vi "HEWH_Ritter_GasMeter.vi"(8 "error in":errorcluster, 11 "Message Queues out":T1) -> (0 "error out":errorcluster)   [LabVIEW 2023]
uses:
  Tenney/support/Message Queue/All Message Queues.ctl
  Tenney/support/Message Queue/Message Cluster.ctl
  Drivers/Ritter Gas Meter/Type Definitions/Ritter Data.ctl
  FVIR and LDO/support/Message Queue/Enqueue Message (Single).vi
  FVIR and LDO/support/Message Queue/Message Queue.lvlib
  Tenney/support/Message Queue/Tenney Message Queue.lvlib
panel:
  out "Loop Count":i32
  in  "Debug":bool
  out "Debug":string[](array[string])
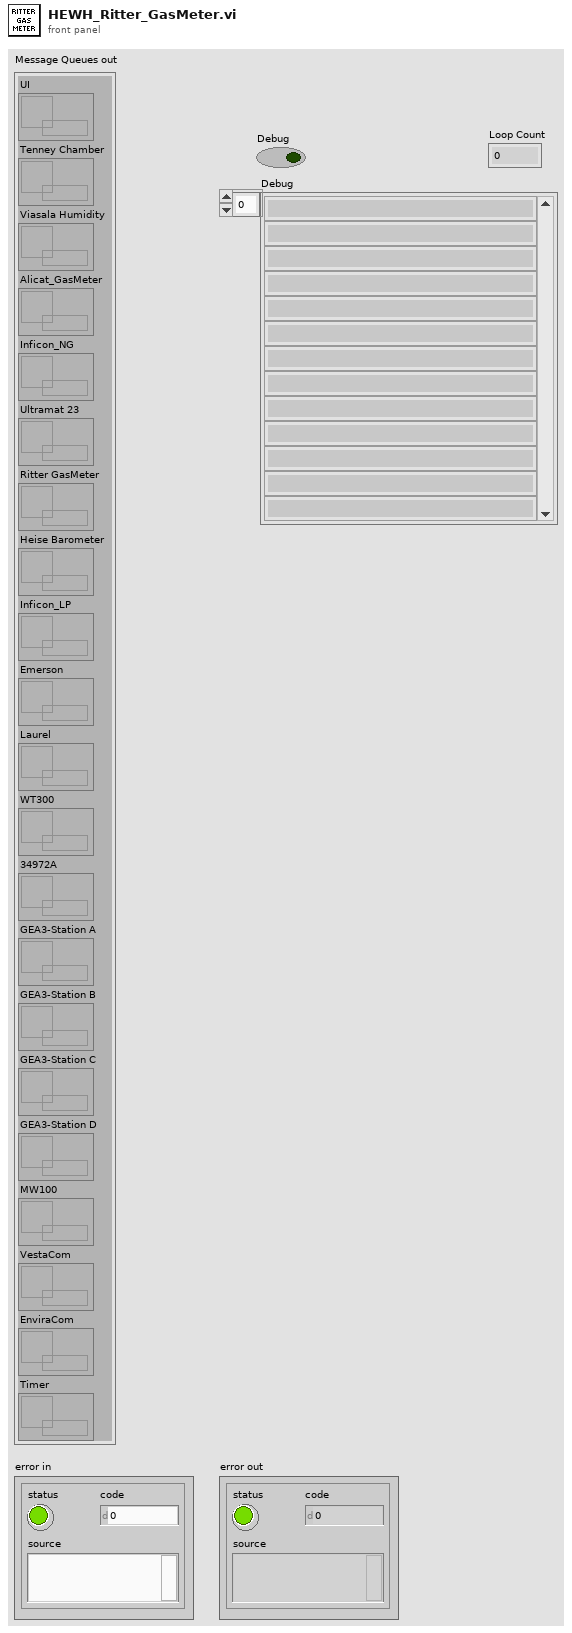
[diagram p1: front panel]
types:
  T1 = typedef "Tenney Message Queue.lvlib/All Message Queues.ctl" = cluster{"UI":refnum<queue>, "Tenney Chamber":refnum<queue>, "Viasala Humidity":refnum<queue>, "Alicat_GasMeter":refnum<queue>, "Inficon_NG":refnum<queue>, "Ultramat 23":refnum<queue>, "Ritter GasMeter":refnum<queue>, "Heise Barometer":refnum<queue>, "Inficon_LP":refnum<queue>, "Emerson":refnum<queue>, "Laurel":refnum<queue>, "WT300":refnum<queue>, "34972A":refnum<queue>, "GEA3-Station A":refnum<queue>, "GEA3-Station B":refnum<queue>, "GEA3-Station C":refnum<queue>, "GEA3-Station D":refnum<queue>, "MW100":refnum<queue>, "VestaCom":refnum<queue>, "EnviraCom":refnum<queue>, "Timer":refnum<queue>}
  T2 = typedef "Ritter Data.ctl" = cluster{"Gas Flow Rate (L/hr)-Uncorrected":dbl, "Totalized Flow (L)--Uncorrected":dbl, "Gas Flow Rate (cuft/hr)-Uncorrected":dbl, "Totalized Flow (cuft)-Uncorrected":dbl, "Gas Temperature (F)":dbl, "Gas Pressure (in WC)":dbl, "Heise Barometric Pressure (inHG)":dbl, "STP Correction Factor":dbl, "Temp Correction Factor":dbl, "Pressure Correction Factor":dbl, "Water Vapor Pressure":dbl, "Gas Flow Rate (cuft/hr)-Corrected":dbl, "Totalized Flow (cuft)-Corrected":dbl, "Gas BTU":dbl, "Gas BTU/hr":dbl}
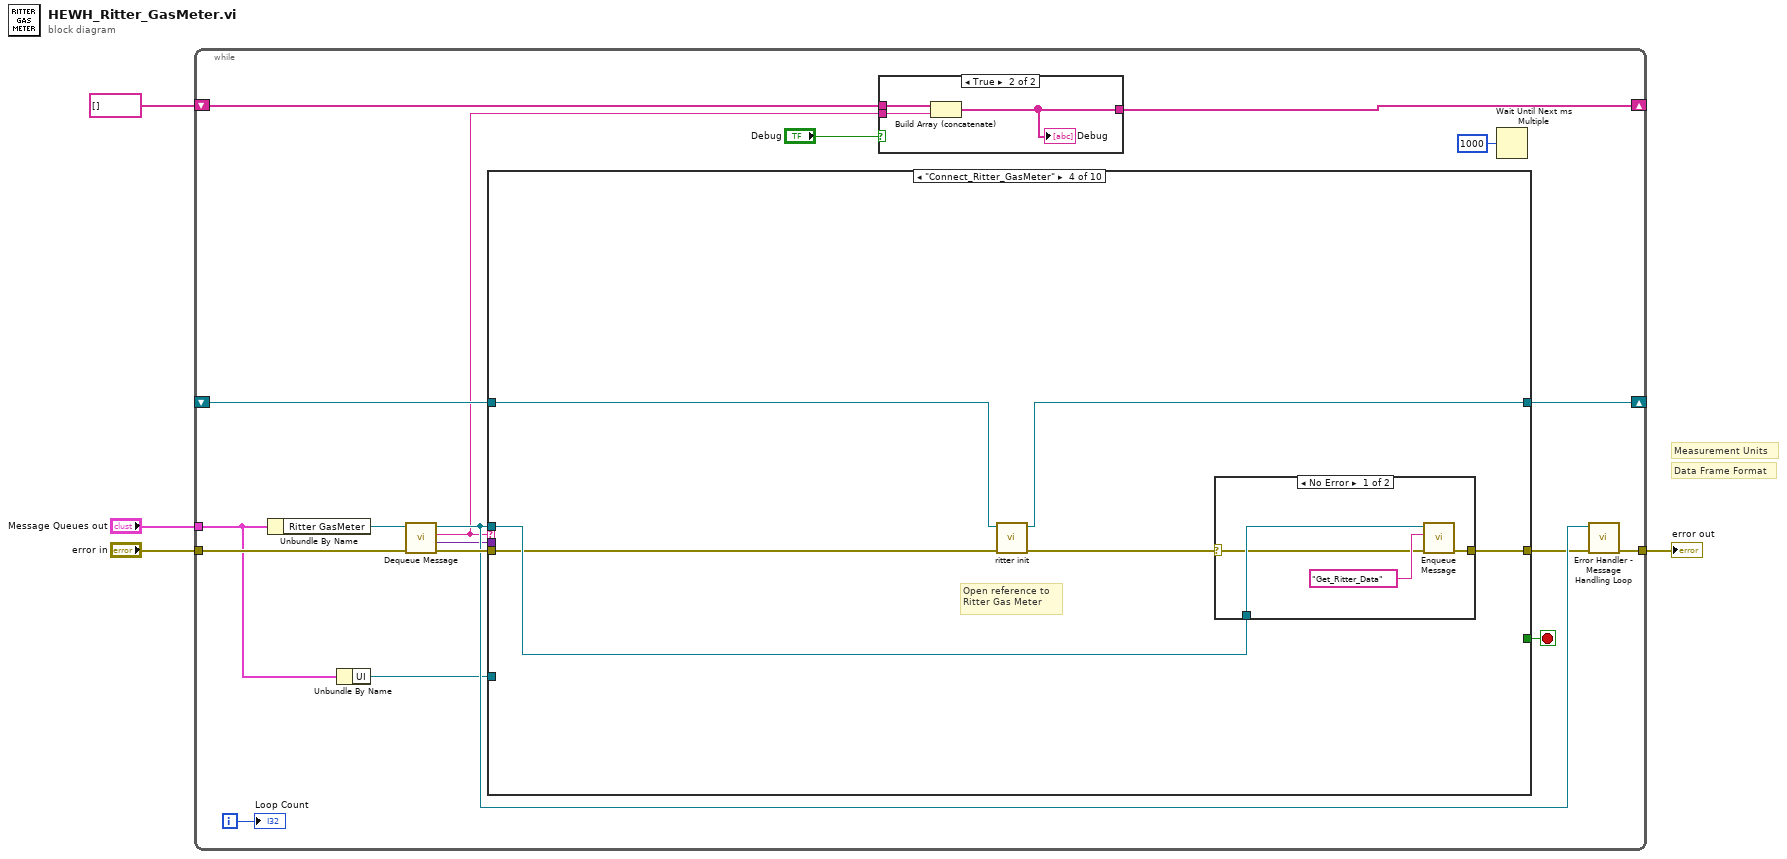
[diagram p0: block diagram]
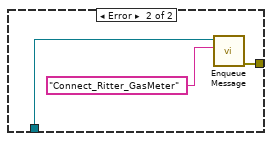
[diagram p6: hidden frame]
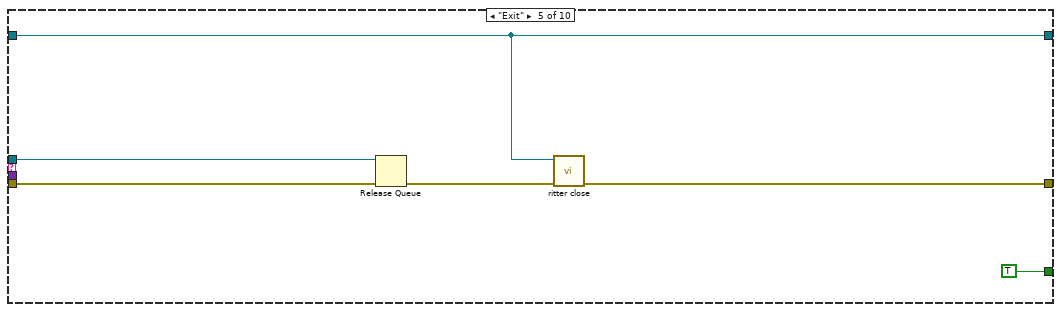
[diagram p7: hidden frame]
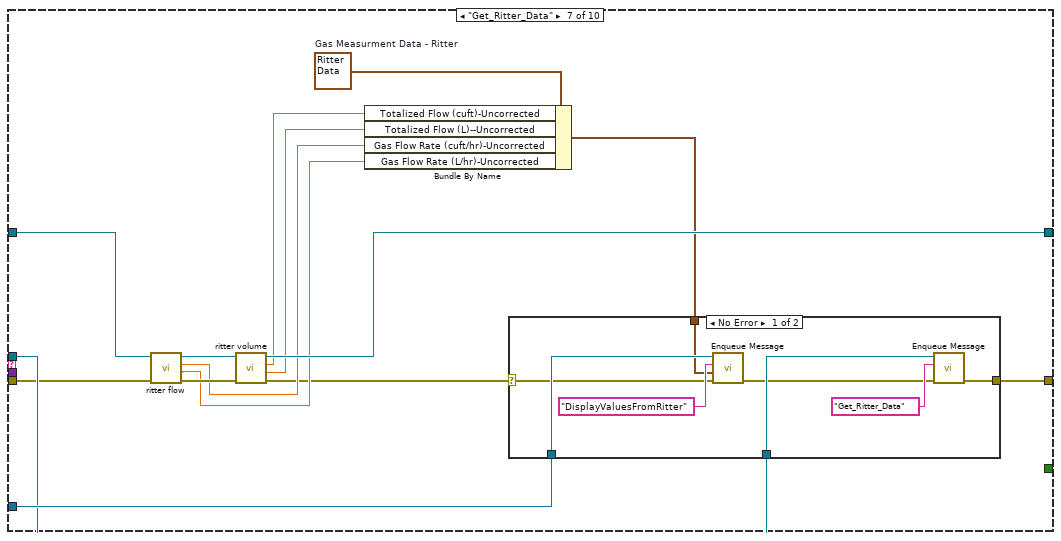
[diagram p9: hidden frame]
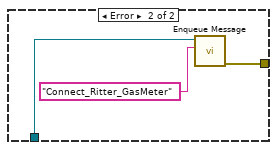
[diagram p10: hidden frame]
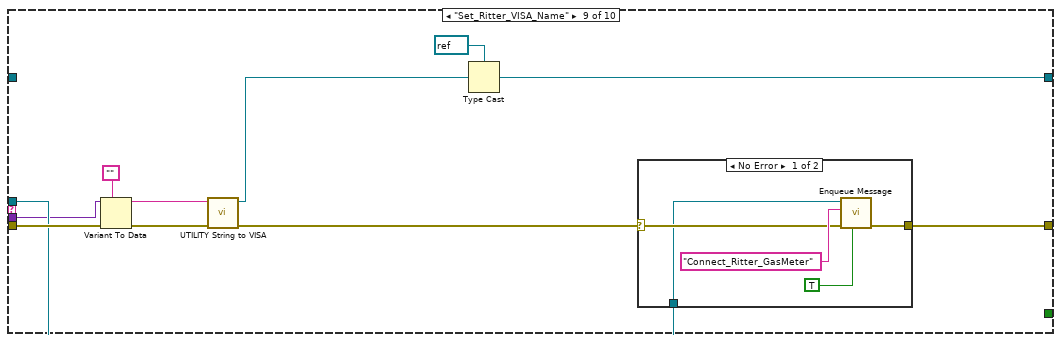
[diagram p12: hidden frame]
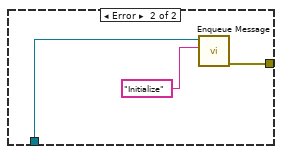
[diagram p13: hidden frame]
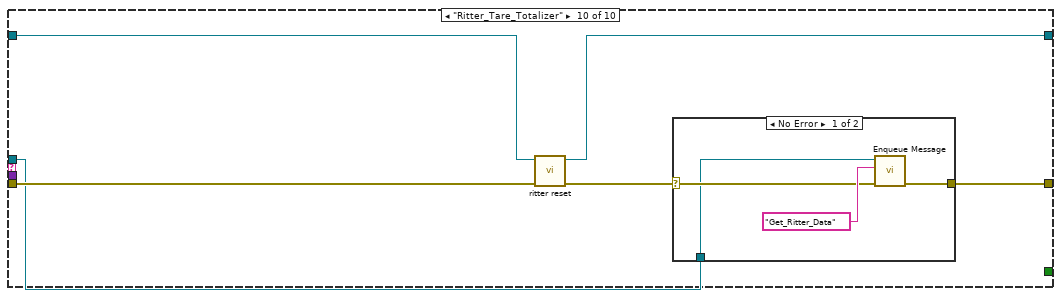
[diagram p14: hidden frame]
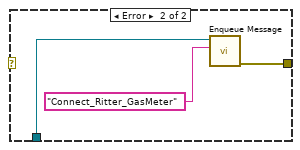
[diagram p15: hidden frame]
diagram:
  # "Data Frame Format"
  # "Measurement Units"
  n1 = while {
    tunnel: "Message Queues out" -> [w12]
    tunnel: "error in" -> [w21]
    tunnel: [w17] -> w3
    shift-right: [w15] -> _
    shift-left: _ -> [w14]
    shift-right: [w8] -> _
    shift-left: string[] [] -> [w9]
    i -> [w5]
    stop <- w19 stop-if-true
    n2 = Unbundle By Name(w12) -> ("Ritter GasMeter"=w22:refnum<queue>)
    n3 = Unbundle By Name(w12) -> ("UI"=w11:refnum<queue>)
    n4 = call "Dequeue Message.vi"("error in (no error)"=w21, "Message Queue"=w22) -> ("error out"=w20:errorcluster, "Message Data"=w6:variant, "Message"=w10:string, "dup Message Queue"=w18:refnum<queue>)  [unwired: 6 in]
    n5 = case shown="\"Connect_Ritter_GasMeter\"" w10 {
      tunnel: w20 -> [w27 w29 w31 w36 w46 w52 w63 w80 w89 w106]
      tunnel: [w27 w29 w31 w38 w48 w52 w67 w80 w87 w102] -> w16
      tunnel: [_ _ _ _ TRUE _ _ _ _ _] -> w19
      tunnel: w18 -> [_ _ _ w37 w50 _ w66 _ w86 w101]
      tunnel: [w28 w30 w32 w35 w47 w53 w61 w81 w82 w104] -> w15
      tunnel: w14 -> [w28 w30 w32 w33 w47 w53 w62 w81 _ w105]
      tunnel: w11 -> [_ _ _ _ _ _ w68 _ _ _]
      tunnel: w6 -> [_ _ _ _ _ _ _ _ w85 _]
      frame "---------- Setup ----------" {
      }
      frame Default {
      }
      frame "Initialize" {
      }
      frame "Connect_Ritter_GasMeter" {
        # "Open reference to \nRitter Gas Meter"
        n6 = call "ritter init.vi"("error in (no error)"=w36, "VISA in"=w33) -> ("error out"=w34:errorcluster, "VISA out"=w35:refnum<visa-resource-name>)  [unwired: 8 in]
        n7 = case shown="No Error" w34 {
          selector: w34 -> [w39 _]
          tunnel: [w41 w44] -> w38
          tunnel: w37 -> [w40 w43]
          frame No Error {
            n8 = call-poly "Enqueue Message.vi"("error in (no error)"=w39, "Message"="Get_Ritter_Data", "Message Queue"=w40) -> ("error out"=w41:errorcluster)  [unwired: 7 in, 1 out]
          }
          frame Error {
            n9 = call-poly "Enqueue Message.vi"("Message"="Connect_Ritter_GasMeter", "Message Queue"=w43) -> ("error out"=w44:errorcluster)  [unwired: 8 in, 1 out]
          }
        }
      }
      frame "Exit" {
        n10 = Release Queue(queue=w50, error in (no error)=w46) -> (error out=w49:errorcluster)  [unwired: 1 in, 2 out]
        n11 = call "ritter close.vi"("error in (no error)"=w49, "VISA in"=w47) -> ("error out"=w48:errorcluster)  [unwired: 9 in]
      }
      frame "---------- Data Collection ----------" {
      }
      frame "Get_Ritter_Data" {
        w60 = T2 {"Gas Flow Rate (L/hr)-Uncorrected"=0.0, "Totalized Flow (L)--Uncorrected"=0.0, "Gas Flow Rate (cuft/hr)-Uncorrected"=0.0, "Totalized Flow (cuft)-Uncorrected"=0.0, "Gas Temperature (F)"=0.0, "Gas Pressure (in WC)"=0.0, "Heise Barometric Pressure (inHG)"=0.0, "STP Correction Factor"=0.0, "Temp Correction Factor"=0.0, "Pressure Correction Factor"=0.0, "Water Vapor Pressure"=0.0, "Gas Flow Rate (cuft/hr)-Corrected"=0.0, "Totalized Flow (cuft)-Corrected"=0.0, "Gas BTU"=0.0, "Gas BTU/hr"=0.0}  # Gas Measurment Data - Ritter
        n12 = call "ritter flow.vi"("error in (no error)"=w63, "VISA in"=w62) -> ("error out"=w64:errorcluster, "flow (ltr/hr)"=w56:dbl, "flow (cuft/hr)"=w57:dbl, "VISA out"=w65:refnum<visa-resource-name>)  [unwired: 6 in]
        n13 = call "ritter volume.vi"("error in (no error)"=w64, "VISA in"=w65) -> ("error out"=w54:errorcluster, "volume (liters)"=w58:dbl, "volume (cuft)"=w59:dbl, "VISA out"=w61:refnum<visa-resource-name>)  [unwired: 6 in]
        n14 = Bundle By Name(cluster=w60, "Totalized Flow (cuft)-Uncorrected"=w59, "Totalized Flow (L)--Uncorrected"=w58, "Gas Flow Rate (cuft/hr)-Uncorrected"=w57, "Gas Flow Rate (L/hr)-Uncorrected"=w56) -> (w55:T2)
        n15 = case shown="No Error" w54 {
          selector: w54 -> [w69 _]
          tunnel: w68 -> [w75 _]
          tunnel: [w74 w78] -> w67
          tunnel: w66 -> [w73 w77]
          tunnel: w55 -> [w72 _]
          frame No Error {
            n16 = call-poly "Enqueue Message.vi"("error in (no error)"=w69, "Message Data"=w72, "Message"="DisplayValuesFromRitter", "Message Queue"=w75) -> ("error out"=w70:errorcluster)  [unwired: 6 in, 1 out]
            n17 = call-poly "Enqueue Message.vi"("error in (no error)"=w70, "Message"="Get_Ritter_Data", "Message Queue"=w73) -> ("error out"=w74:errorcluster)  [unwired: 7 in, 1 out]
          }
          frame Error {
            n18 = call-poly "Enqueue Message.vi"("Message"="Connect_Ritter_GasMeter", "Message Queue"=w77) -> ("error out"=w78:errorcluster)  [unwired: 8 in, 1 out]
          }
        }
      }
      frame "---------- Events ----------" {
      }
      frame "Set_Ritter_VISA_Name" {
        n19 = Variant To Data(error in=w89, type="", Variant=w85) -> (data=w92:string, error out=w91:errorcluster)
        n20 = call "UTILITY String to VISA.vi"("error in (no error)"=w91, "VISA Name"=w92) -> ("error out"=w88:errorcluster, "VISA resource name out"=w83:refnum<visa-resource-name>)  [unwired: 8 in]
        n21 = Type Cast(type=refnum<visa-resource-name> refnum ("VISA out"), x=w83) -> (*(type *) &x=w82:refnum<visa-resource-name>)
        n22 = case shown="No Error" w88 {
          selector: w88 -> [w95 _]
          tunnel: [w94 w99] -> w87
          tunnel: w86 -> [w93 w98]
          frame No Error {
            n23 = call-poly "Enqueue Message.vi"("Priority Message? (F)"=TRUE, "error in (no error)"=w95, "Message"="Connect_Ritter_GasMeter", "Message Queue"=w93) -> ("error out"=w94:errorcluster)  [unwired: 6 in, 1 out]
          }
          frame Error {
            n24 = call-poly "Enqueue Message.vi"("Message"="Initialize", "Message Queue"=w98) -> ("error out"=w99:errorcluster)  [unwired: 8 in, 1 out]
          }
        }
      }
      frame "Ritter_Tare_Totalizer" {
        n25 = call "ritter reset.vi"("error in (no error)"=w106, "VISA in"=w105) -> ("error out"=w103:errorcluster, "VISA out"=w104:refnum<visa-resource-name>)  [unwired: 8 in]
        n26 = case shown="No Error" w103 {
          selector: w103 -> [w109 _]
          tunnel: [w108 w112] -> w102
          tunnel: w101 -> [w107 w111]
          frame No Error {
            n27 = call-poly "Enqueue Message.vi"("error in (no error)"=w109, "Message"="Get_Ritter_Data", "Message Queue"=w107) -> ("error out"=w108:errorcluster)  [unwired: 7 in, 1 out]
          }
          frame Error {
            n28 = call-poly "Enqueue Message.vi"("Message"="Connect_Ritter_GasMeter", "Message Queue"=w111) -> ("error out"=w112:errorcluster)  [unwired: 8 in, 1 out]
          }
        }
      }
    }
    n29 = case shown="True" "Debug" {
      tunnel: w10 -> [_ w26]
      tunnel: w9 -> [w23 w25]
      tunnel: [w23 w24] -> w8
      frame False {
      }
      frame True {
        n30 = Build Array (concatenate)(w25, w26) -> (w24:string[])
        "Debug" <- w24
      }
    }
    n31 = Wait Until Next ms Multiple(millisecond multiple=u32 1000) -> ()  [unwired: 1 out]
    n32 = call "Error Handler - Message Handling Loop.vi"("error in (no error)"=w16, "Message Queue"=w18) -> ("dup error in"=w17:errorcluster)  [unwired: 8 in, 1 out]
    "Loop Count" <- w5
  }
  "error out" <- w3
